vi "InitGraphConfig.vi"(0 "Interface en entrée":refnum<class "Interface.lvclass"> caption="DNL_LabVIEW Object in", 1 "GraphClosedRef":refnum<vi>, 3 "PlotChange":refnum<vi>, 5 "Graph_FA":refnum<vi>[](array[refnum]), 7 "PanRef":refnum<vi>, 9 "ListboxRef":refnum<vi>, 11 "error in (no error)":errorcluster caption="entrée d'erreur (pas d'erreur)") -> (4 "Interface en sortie":refnum<class "Interface.lvclass"> caption="DNL_LabVIEW Object out", 6 "Graph Event":refnum<user-event>, 15 "error out":errorcluster caption="sortie d'erreur")   [LabVIEW 2010, in "Interface.lvclass"]
uses:
  Interface.lvclass
  Interface.lvclass/Interface.ctl
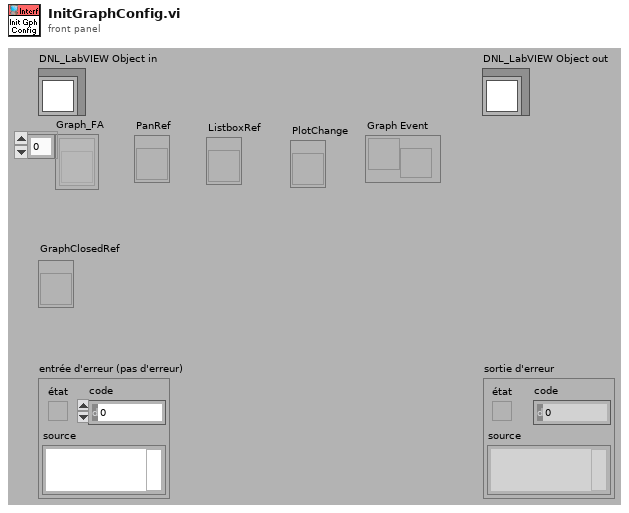
[diagram p1: front panel]
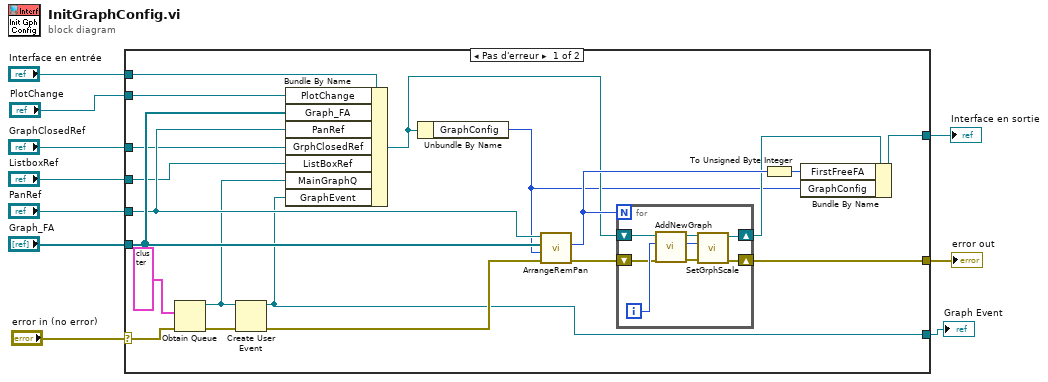
[diagram p0: block diagram]
diagram:
  n1 = case shown="Pas d'erreur" "error in (no error)" {
    selector: "error in (no error)" -> [w14 w40]
    tunnel: [w25 w40] -> w9
    tunnel: [w29 w39] -> w7
    tunnel: "Interface en entrée" -> [w30 w39]
    tunnel: "Graph_FA" -> [w24 _]
    tunnel: "PanRef" -> [w22 _]
    tunnel: "GraphClosedRef" -> [w21 _]
    tunnel: "ListboxRef" -> [w20 _]
    tunnel: "PlotChange" -> [w19 _]
    tunnel: [w11 _] -> w1
    frame No Error {
      n2 = Obtain Queue(element data type=cluster{"Message":string, "Data":variant, i32} {"Message"="", "Data"=variant, 0} ("ClassQueue"), error in (no error)=w14) -> (queue out=w12:refnum<queue>, error out=w15:errorcluster)  [unwired: 3 in, 1 out]
      n3 = Create User Event(user event datatype=w12, error in=w15) -> (user event=w11:refnum<user-event>, error out=w13:errorcluster)
      n4 = Bundle By Name(cluster=w30, "PlotChange"=w19, "Graph_FA"=w24, "PanRef"=w22, "GrphClosedRef"=w21, "ListBoxRef"=w20, "MainGraphQ"=w12, "GraphEvent"=w11) -> (w18:refnum<class "Interface.lvclass">)
      n5 = Unbundle By Name(w18) -> ("GraphConfig"=w17:i32)
      n6 = call "ArrangeRemPan.vi"("error in (no error)"=w13, "Configuration"=w17, "FARefArr"=w24, "PanRef"=w22) -> ("error out"=w27:errorcluster, "GraphCount"=w26:i32)  [unwired: 5 in, 1 out]
      n7 = for {
        N: w26 -> [_]
        shift-right: [w33] -> w25
        shift-left: w27 -> [w37]
        shift-right: [w34] -> w23
        shift-left: w18 -> [w36]
        i -> [w38]
        n8 = call "AddNewGraph.vi"("error in (no error)"=w37, "FAIndex"=w38, "Interface en entrée"=w36) -> ("error out"=w32:errorcluster, "NewGraphInd"=w31:i32, "Interface en sortie"=w35:refnum<class "Interface.lvclass">)  [unwired: 6 in]
        n9 = call "SetGrphScale.vi"("error in (no error)"=w32, "GraphIndex"=w31, "Interface en entrée"=w35) -> ("error out"=w33:errorcluster, "Interface en sortie"=w34:refnum<class "Interface.lvclass">)  [unwired: 7 in]
      }
      n10 = To Unsigned Byte Integer(number=w26) -> (unsigned 8bit integer=w28:u8)
      n11 = Bundle By Name(cluster=w23, "FirstFreeFA"=w28, "GraphConfig"=w17) -> (w29:refnum<class "Interface.lvclass">)
    }
    frame Error {
    }
  }
  "error out" <- w9
  "Interface en sortie" <- w7
  "Graph Event" <- w1
